vi "FTW-Endpoint-Destroy.vi"(0 "FTW Endpoint":refnum<class "FTW-Endpoint.lvclass">, 5 "Force Destroy":bool, 11 "error in":errorcluster) -> (15 "error out":errorcluster)   [LabVIEW 2013, in "FTW-Endpoint.lvclass"]
uses:
  FTW-Endpoint.lvclass
  FTW-Endpoint.lvclass/FTW-Endpoint.ctl
panel:
  # "Inputs"
  # "Outputs"
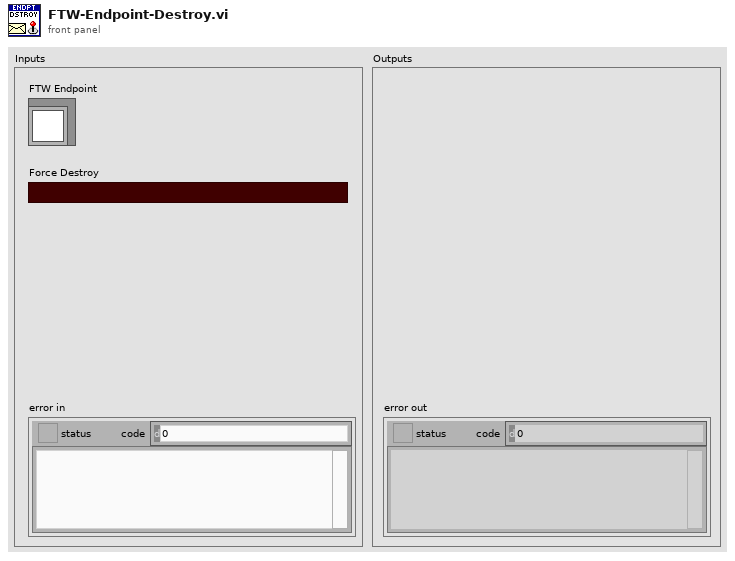
[diagram p1: front panel]
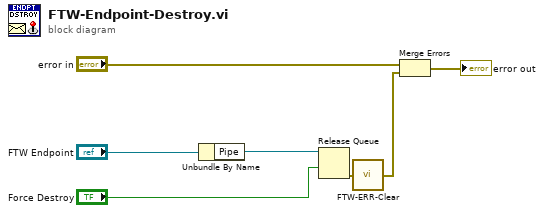
[diagram p0: block diagram]
diagram:
  n1 = Unbundle By Name("FTW Endpoint") -> ("Pipe"=w6:refnum<queue>)
  n2 = Release Queue(queue=w6, force destroy? (F)="Force Destroy") -> (error out=w2:errorcluster)  [unwired: 1 in, 2 out]
  n3 = call "FTW-ERR-Clear.vi"("error to snuff"=w2) -> ("no error"=w1:errorcluster)
  n4 = Merge Errors("error in", w1) -> (→"error out":errorcluster)
